vi "Write Find Fiducials.vi"(8 "error in (no error)":errorcluster, 10 "Find Fiducials":T1, 11 "Gluing Procedure in":refnum<class "Gluing Procedure.lvclass">) -> (0 "error out":errorcluster, 3 "Gluing Procedure out":refnum<class "Gluing Procedure.lvclass">)   [LabVIEW 2017, in "Gluing Procedure.lvclass"]
uses:
  Gluing Procedure.lvclass
  Shared Components/Vec3d Class/Vec3d Class.lvclass
  <vilib>/vision/Image Controls.llb/IMAQ Image.ctl
  Shared Components/Utils/Type Definitions/Physical Image.ctl
  Shared Components/Utils/Type Definitions/Fiducial with Source.ctl
  Shared Components/Utils/Type Definitions/Fiducial Image.ctl
  Shared Components/Utils/Type Definitions/Part Fiducials.ctl
  Type Definitions/Inspect Fuducials.ctl
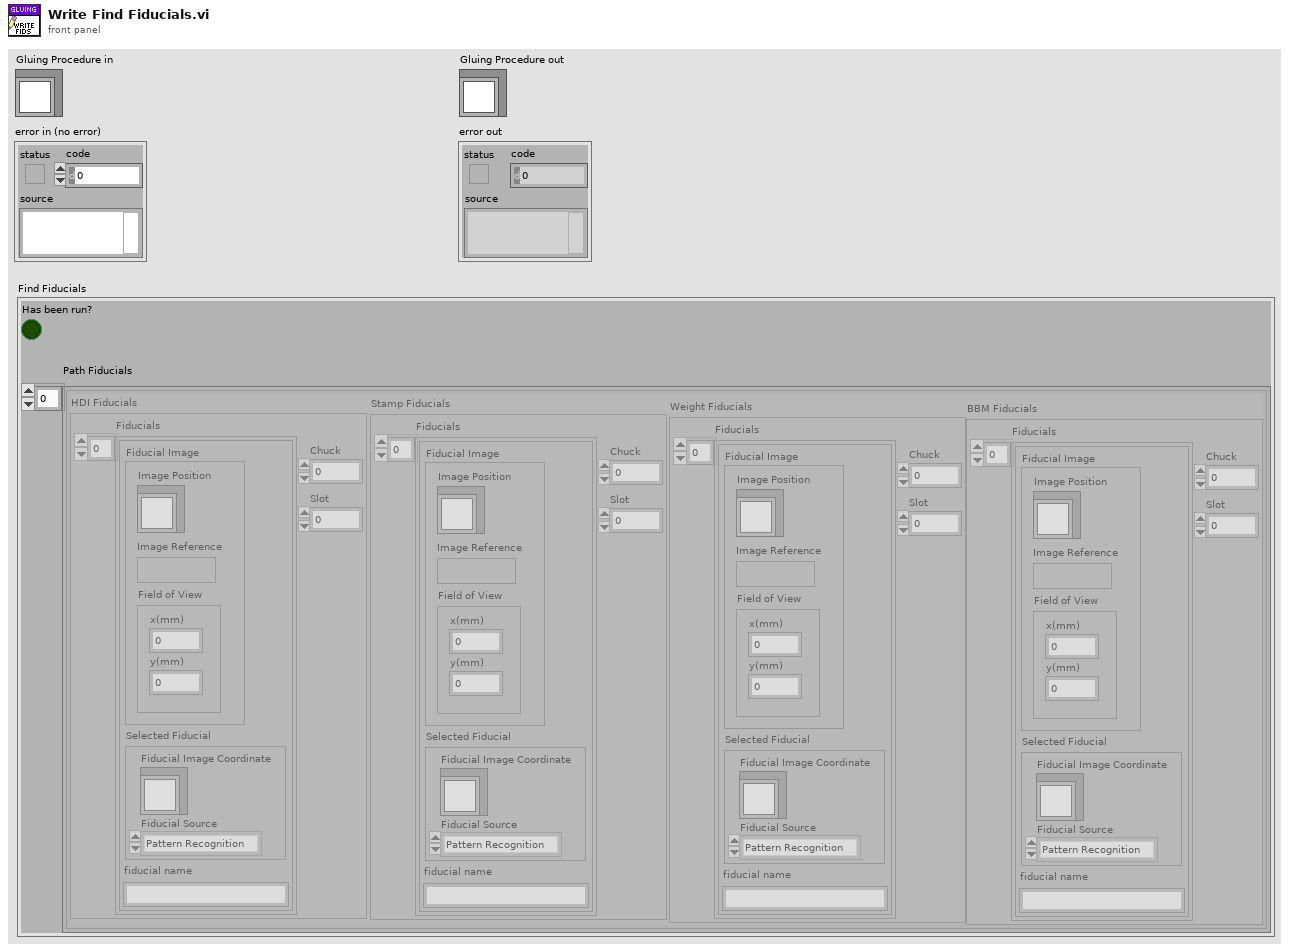
[diagram p1: front panel]
types:
  T1 = typedef "Inspect Fuducials.ctl" = cluster{"Path Fiducials":cluster{"HDI Fiducials":T2, "Stamp Fiducials":T2, "Weight Fiducials":T2, "BBM Fiducials":T2}[], "Has been run?":bool}
  T2 = typedef "Part Fiducials.ctl" = cluster{"Fiducials":T3[], "Chuck":i32, "Slot":i32}
  T3 = typedef "Fiducial Image.ctl" = cluster{"Fiducial Image":T4, "Selected Fiducial":T6, "fiducial name":string}
  T4 = typedef "Physical Image.ctl" = cluster{"Image Position":refnum<class "Vec3d Class.lvclass">, "Image Reference":T5, "Field of View":cluster{"x(mm)":dbl, "y(mm)":dbl}}
  T5 = typedef "IMAQ Image.ctl" = refnum<image>
  T6 = typedef "Fiducial with Source.ctl" = cluster{"Fiducial Image Coordinate":refnum<class "Vec3d Class.lvclass">, "Fiducial Source":enum16{"Pattern Recognition", "User", "Error", "Default"}}
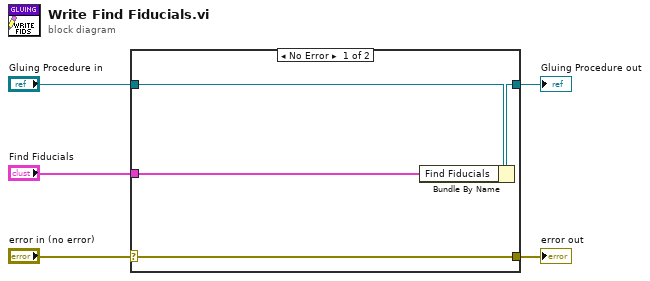
[diagram p0: block diagram]
diagram:
  n1 = case shown="No Error" "error in (no error)" {
    selector: "error in (no error)" -> [w9 w10]
    tunnel: [w9 w10] -> w4
    tunnel: [w7 w11] -> w2
    tunnel: "Gluing Procedure in" -> [w8 w11]
    tunnel: "Find Fiducials" -> [w6 _]
    frame No Error {
      n2 = Bundle By Name(cluster=w8, "Find Fiducials"=w6) -> (w7:refnum<class "Gluing Procedure.lvclass">)
    }
    frame Error {
    }
  }
  "error out" <- w4
  "Gluing Procedure out" <- w2
